vi "PicoScope5000aGetTriggerInfo.vi"(0 "handle in":i16, 5 "Rapid Block Acquisition Settings":T2 {"toSegmentIndex" format="%.4p"; "fromSegmentIndex" format="%.4p"}, 9 "Sample Rate":sgl, 11 "error in":errorcluster) -> (4 "handle out":i16, 6 "Trigger Info":T1(array[cluster]), 10 "Trigger Offsets":cluster{u64, sgl}[](array[cluster]) {"?" format="%#_5p"}, 15 "error out":errorcluster)   [LabVIEW 2010]
doc: "This VI gets a set of Trigger time Info structures and calculates times deltas, captured using rapid block mode."
uses:
  ps5000a.dll
  shared/Segment Range.ctl
panel:
  out "Number of Captures":u32=1
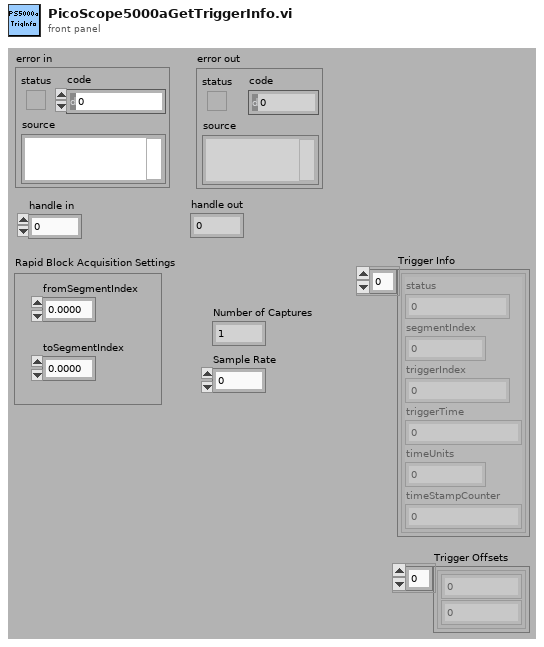
[diagram p1: front panel]
types:
  T1 = cluster{"status":u32, "segmentIndex":u32, "triggerIndex":u32, "triggerTime":i64, "timeUnits":i16, "timeStampCounter":u64}[]
  T2 = typedef "Segment Range.ctl" = cluster{"fromSegmentIndex":u64, "toSegmentIndex":u64}
  T3 = cluster{"status":u32, "segmentIndex":u32, "triggerIndex":u32, "triggerTime":i64, "timeUnits":i16, "reserved0":i16, "timeStampCounter":u64}
  T4 = cluster{"status":bool, "code":u32, "source":string}
  T5 = cluster{"status":u32, "segmentIndex":u32, "triggerIndex":u32, "triggerTime":i64, "timeUnits":i16, "timeStampCounter":u64}
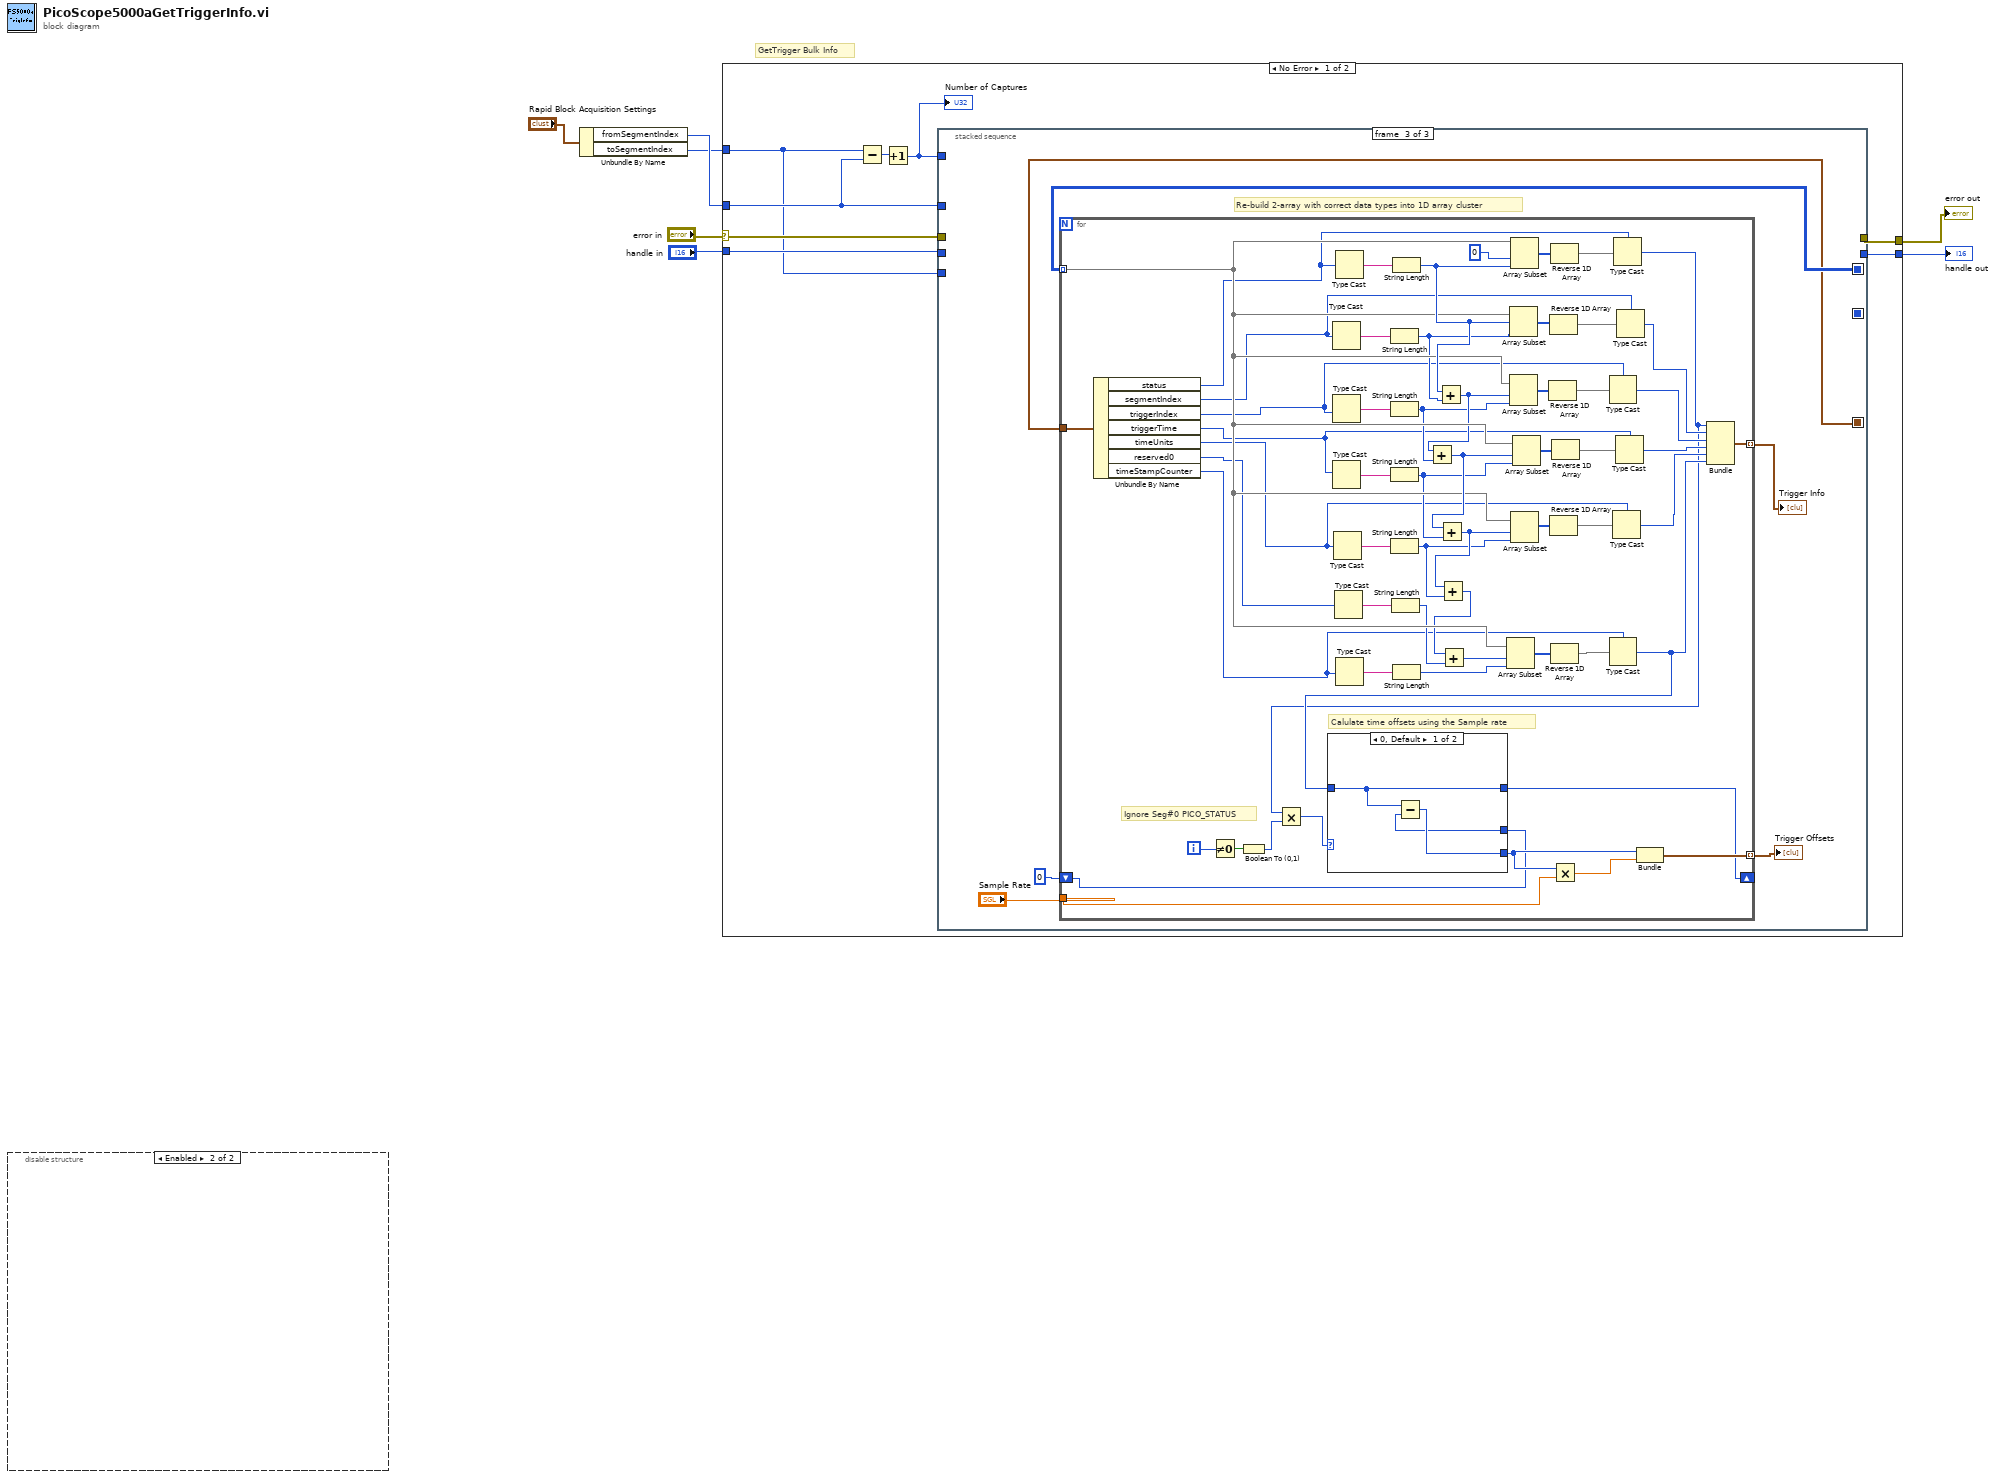
[diagram p0: block diagram]
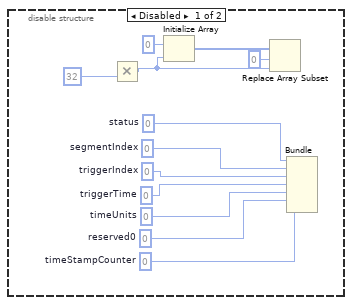
[diagram p2: hidden frame]
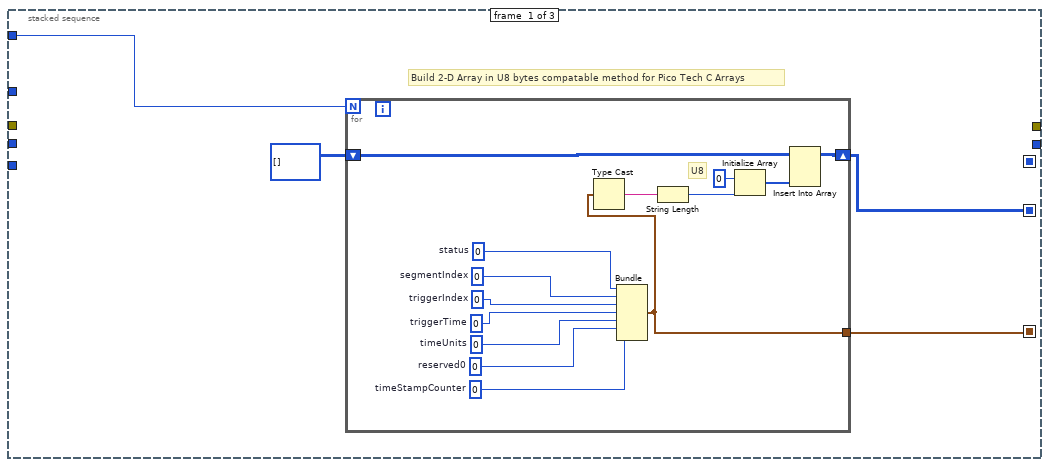
[diagram p3: hidden frame]
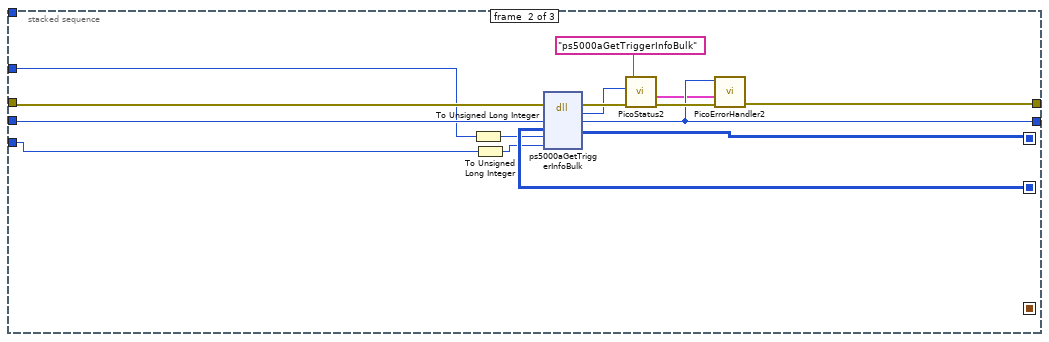
[diagram p4: hidden frame]
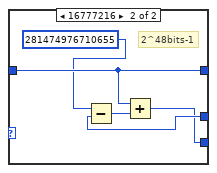
[diagram p5: hidden frame]
diagram:
  # "GetTrigger Bulk Info"
  n1 = disable-structure shown="Enabled" {
    frame Disabled {
      w15 = u64 0  # timeStampCounter
      w13 = i16 0  # reserved0
      w14 = i16 0  # timeUnits
      w16 = i64 0  # triggerTime
      w17 = u32 0  # triggerIndex
      w18 = u32 0  # segmentIndex
      w19 = u32 0  # status
      n2 = Multiply(y=u32 32) -> (x*y=w11:u32)  [unwired: 1 in]
      n3 = Initialize Array(u8 0 ("element"), w11) -> (w12:u8[])
      n4 = Replace Array Subset(array=w12, new element=w11, index=0) -> ()  [unwired: 1 out]
      n5 = Bundle("status"=w19, "segmentIndex"=w18, "triggerIndex"=w17, "triggerTime"=w16, "timeUnits"=w14, "reserved0"=w13, "timeStampCounter"=w15) -> ()  [unwired: 1 in, 1 out]
    }
    frame Enabled {
    }
  }
  n6 = Unbundle By Name("Rapid Block Acquisition Settings") -> ("fromSegmentIndex"=w3:u64, "toSegmentIndex"=w2:u64)
  n7 = case shown="No Error" "error in" {
    selector: "error in" -> [w27 w135]
    tunnel: [w25 w135] -> w1
    tunnel: "handle in" -> [w26 w134]
    tunnel: [w24 w134] -> w5
    tunnel: w2 -> [w21 _]
    tunnel: w3 -> [w22 _]
    frame No Error {
      n8 = Subtract(x=w21, y=w22) -> (x-y=w23:u64)
      n9 = Increment(x=w23) -> (x+1=w20:u64)
      "Number of Captures" <- w20
      n10 = stacked-sequence {
        seq-local: [w29 _ _] -> [_ w56 _]
        seq-local: [w28 _ _] -> [_ w54 _]
        seq-local: [_ w55 _] -> [_ _ w67]
        seq-local: [_ w54 _] -> [_ _ w63]
        tunnel: w20 -> [w31 _ _]
        tunnel: w27 -> [_ w58 _]
        tunnel: w26 -> [_ w57 _]
        tunnel: w22 -> [_ w53 _]
        tunnel: w21 -> [_ w50 _]
        tunnel: [_ w46 _] -> w25
        tunnel: [_ w48 _] -> w24
        frame #0 {
          # "Build 2-D Array in U8 bytes compatable method for Pico Tech C Arrays"
          n11 = for {
            N: w31 -> [_]
            shift-right: [w33] -> w29
            shift-left: u8[][] [] -> [w34]
            tunnel: [w32] -> w28
            w41 = u64 0  # timeStampCounter
            w39 = i16 0  # reserved0
            w40 = i16 0  # timeUnits
            w42 = i64 0  # triggerTime
            w43 = u32 0  # triggerIndex
            w44 = u32 0  # segmentIndex
            w45 = u32 0  # status
            # "U8"
            n12 = Bundle("status"=w45, "segmentIndex"=w44, "triggerIndex"=w43, "triggerTime"=w42, "timeUnits"=w40, "reserved0"=w39, "timeStampCounter"=w41) -> (w32:T3)  [unwired: 1 in]
            n13 = Type Cast(x=w32) -> (*(type *) &x=w38:string)  [unwired: 1 in]
            n14 = String Length(string=w38) -> (length=w36:i32)
            n15 = Initialize Array(u8 0 ("element"), w36) -> (w35:u8[])
            n16 = Insert Into Array(array=w34, new element=w35) -> (w33:u8[][])  [unwired: 2 in]
          }
        }
        frame #1 {
          n17 = To Unsigned Long Integer(number=w53) -> (unsigned 32bit integer=w52:u32)
          n18 = To Unsigned Long Integer(number=w50) -> (unsigned 32bit integer=w51:u32)
          n19 = dll-call lib="ps5000a.dll" fn="ps5000aGetTriggerInfoBulk" ("ps3000.dll:_ps3000_open_unit@0")(error in=w58, "handle"=w57, "triggerInfo"=w56, "fromSegmentIndex"=w52, "toSegmentIndex"=w51) -> (error out=w61:errorcluster, "PICO_STATUS"=w60:u32, "handle"=w48:i16, "triggerInfo"=w55:u8[][])  [unwired: 4 in, 1 out]
          n20 = call "PicoStatus2.vi"("PICO source"="ps5000aGetTriggerInfoBulk" ("source"), "Error in"=w61, "PICO STATUS"=w60) -> ("error out"=w49:errorcluster, "PICO_STATUS out"=w47:T4)  [unwired: 5 in]
          n21 = call "PicoErrorHandler2.vi"("error in (no error)"=w49, "PICO_STATUS in"=w47, "handle In"=w48) -> ("error out"=w46:errorcluster)  [unwired: 8 in]
        }
        frame #2 {
          # "Re-build 2-array with correct data types into 1D array cluster"
          n22 = for {
            tunnel: w67 -> [w89] mode=indexing
            tunnel: [w122] -> w66 mode=indexing
            tunnel: [w107] -> w65 mode=indexing
            tunnel: "Sample Rate" -> [w106]
            tunnel: w63 -> [w81]
            shift-right: [w70] -> _
            shift-left: u64 0 ("timeStampCounter") -> [w71]
            i -> [w108]
            # "Calulate time offsets using the Sample rate"
            # "Ignore Seg#0 PICO_STATUS"
            n23 = Unbundle By Name(w81) -> ("status"=w80:u32, "segmentIndex"=w79:u32, "triggerIndex"=w74:u32, "triggerTime"=w75:i64, "timeUnits"=w76:i16, "reserved0"=w77:i16, "timeStampCounter"=w78:u64)
            n24 = Not Equal To 0?(x=w108) -> (x != 0?=w73:bool)
            n25 = Boolean To (0,1)(Boolean=w73) -> (0, 1=w72:i16)
            n26 = Type Cast(x=w79) -> (*(type *) &x=w102:string)  [unwired: 1 in]
            n27 = Type Cast(x=w74) -> (*(type *) &x=w101:string)  [unwired: 1 in]
            n28 = Type Cast(x=w75) -> (*(type *) &x=w100:string)  [unwired: 1 in]
            n29 = Type Cast(x=w76) -> (*(type *) &x=w99:string)  [unwired: 1 in]
            n30 = Type Cast(x=w77) -> (*(type *) &x=w98:string)  [unwired: 1 in]
            n31 = Type Cast(x=w80) -> (*(type *) &x=w103:string)  [unwired: 1 in]
            n32 = Type Cast(x=w78) -> (*(type *) &x=w93:string)  [unwired: 1 in]
            n33 = String Length(string=w102) -> (length=w87:i32)
            n34 = String Length(string=w101) -> (length=w85:i32)
            n35 = String Length(string=w100) -> (length=w84:i32)
            n36 = String Length(string=w99) -> (length=w83:i32)
            n37 = String Length(string=w98) -> (length=w82:i32)
            n38 = String Length(string=w103) -> (length=w94:i32)
            n39 = String Length(string=w93) -> (length=w91:i32)
            n40 = Add(x=w94, y=w87) -> (x+y=w86:i32)
            n41 = Add(x=w86, y=w85) -> (x+y=w97:i32)
            n42 = Add(x=w97, y=w84) -> (x+y=w96:i32)
            n43 = Add(x=w96, y=w83) -> (x+y=w88:i32)
            n44 = Add(x=w88, y=w82) -> (x+y=w92:i32)
            n45 = Array Subset(array=w89, index=w92, length=w91) -> (w90:u8[])
            n46 = Array Subset(array=w89, index=w94, length=w87) -> (w121:u8[])
            n47 = Array Subset(array=w89, index=w86, length=w85) -> (w116:u8[])
            n48 = Array Subset(array=w89, index=0, length=w94) -> (w119:u8[])
            n49 = Array Subset(array=w89, index=w96, length=w83) -> (w113:u8[])
            n50 = Array Subset(array=w89, index=w97, length=w84) -> (w115:u8[])
            n51 = Reverse 1D Array(array=w116) -> (reversed array=w117:u8[])
            n52 = Reverse 1D Array(array=w121) -> (reversed array=w120:u8[])
            n53 = Reverse 1D Array(array=w113) -> (reversed array=w112:u8[])
            n54 = Reverse 1D Array(array=w119) -> (reversed array=w118:u8[])
            n55 = Reverse 1D Array(array=w90) -> (reversed array=w111:u8[])
            n56 = Reverse 1D Array(array=w115) -> (reversed array=w114:u8[])
            n57 = Type Cast(type=w74, x=w117) -> (*(type *) &x=w125:u32)
            n58 = Type Cast(type=w78, x=w111) -> (*(type *) &x=w109:u64)
            n59 = Type Cast(type=w76, x=w112) -> (*(type *) &x=w123:i16)
            n60 = Type Cast(type=w80, x=w118) -> (*(type *) &x=w69:u32)
            n61 = Multiply(x=w69, y=w72) -> (x*y=w68:u32)
            n62 = case shown="0, Default" w68 {
              tunnel: w109 -> [w127 w131]
              tunnel: [w127 w131] -> w70
              tunnel: w71 -> [w126 w133]
              tunnel: [w128 w129] -> w105
              frame 0, Default {
                n63 = Subtract(x=w127, y=w126) -> (x-y=w128:u64)
              }
              frame 16777216 {
                # "2^48bits-1"
                n64 = Subtract(x=u64 281474976710655, y=w133) -> (x-y=w132:u64)
                n65 = Add(x=w131, y=w132) -> (x+y=w129:u64)
              }
            }
            n66 = Multiply(x=w105, y=w106) -> (x*y=w104:sgl)
            n67 = Type Cast(type=w75, x=w114) -> (*(type *) &x=w124:i64)
            n68 = Type Cast(type=w79, x=w120) -> (*(type *) &x=w110:u32)
            n69 = Bundle(w105, w104) -> (w107:cluster{u64, sgl})  [unwired: 1 in]
            n70 = Bundle("status"=w69, "segmentIndex"=w110, "triggerIndex"=w125, "triggerTime"=w124, "timeUnits"=w123, "timeStampCounter"=w109) -> (w122:T5)  [unwired: 1 in]
          }
          "Trigger Info" <- w66
          "Trigger Offsets" <- w65
        }
      }
    }
    frame Error {
    }
  }
  "handle out" <- w5
  "error out" <- w1
